vi "SmoothPath.vi"(9 "enemy_robots":T1[](array[typedef]), 10 "Path":dbl[][](array[numeric])) -> (2 "SmoothPath":dbl[][](array[numeric]))   [LabVIEW 2016]
uses:
  Core/AI Robot.ctl
  Intel/Functions Enum.ctl
  Intel/AttackerStates.ctl
  <vilib>/Analysis/_algsub.llb/Real Vector Norm.vi
  <vilib>/Analysis/baseanly.llb/Real Dot Product.vi
  <vilib>/Analysis/NI_AALBase.lvlib
  <vilib>/Analysis/NI_AALPro.lvlib
panel:
  out "y":dbl
  out "x":dbl
  out "Goal":dbl[](array[numeric])
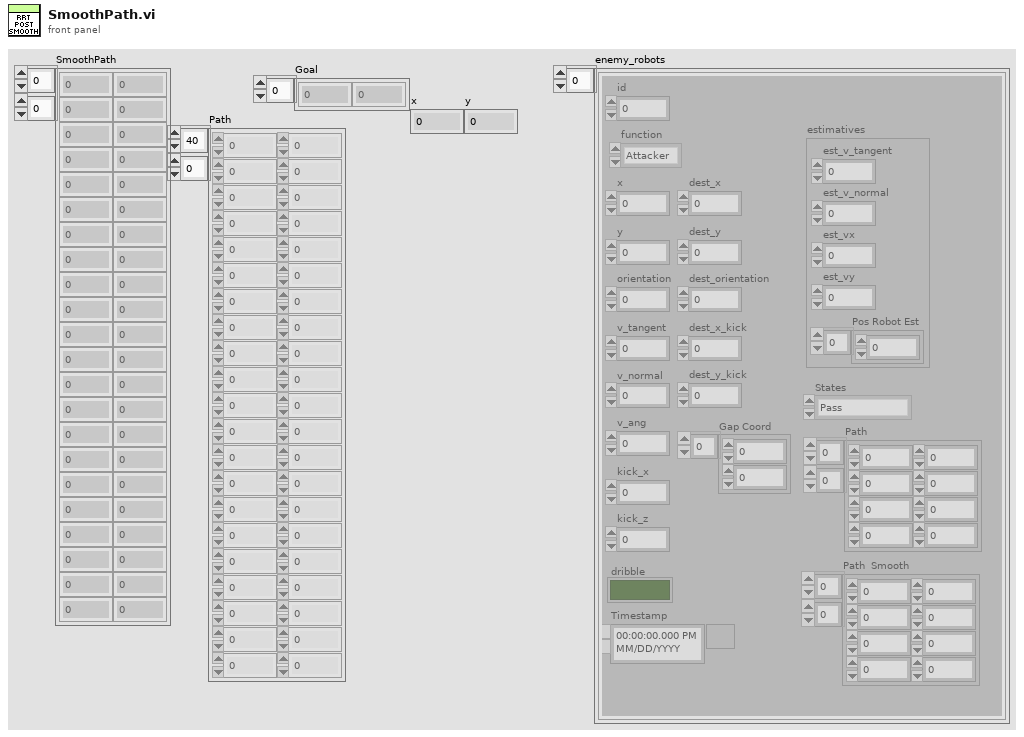
[diagram p1: front panel]
types:
  T1 = typedef "AI Robot.ctl" = cluster{"id":u32, "function":T2, "x":dbl, "y":dbl, "orientation":dbl, "v_tangent":dbl, "v_normal":dbl, "v_ang":dbl, "kick_x":dbl, "kick_z":dbl, "dribble":bool, "Timestamp":timestamp, "dest_x":dbl, "dest_y":dbl, "dest_orientation":dbl, "estimatives":cluster{"est_v_tangent":dbl, "est_v_normal":dbl, "est_vx":dbl, "est_vy":dbl, "Pos Robot Est":dbl[]}, "dest_x_kick":dbl, "dest_y_kick":dbl, "Gap Coord":dbl[], "States":T3, "Path ":dbl[][], "Path  Smooth":dbl[][]}
  T2 = typedef "Functions Enum.ctl" = enum16{"Attacker", "Goalie", "Defender", "Striker", "Goto 0", "Dummy", "Kicker", "ZigZag"}
  T3 = typedef "AttackerStates.ctl" = enum16{"Pass", "GoToTangent", "BallGetting", "GoToKick", ""}
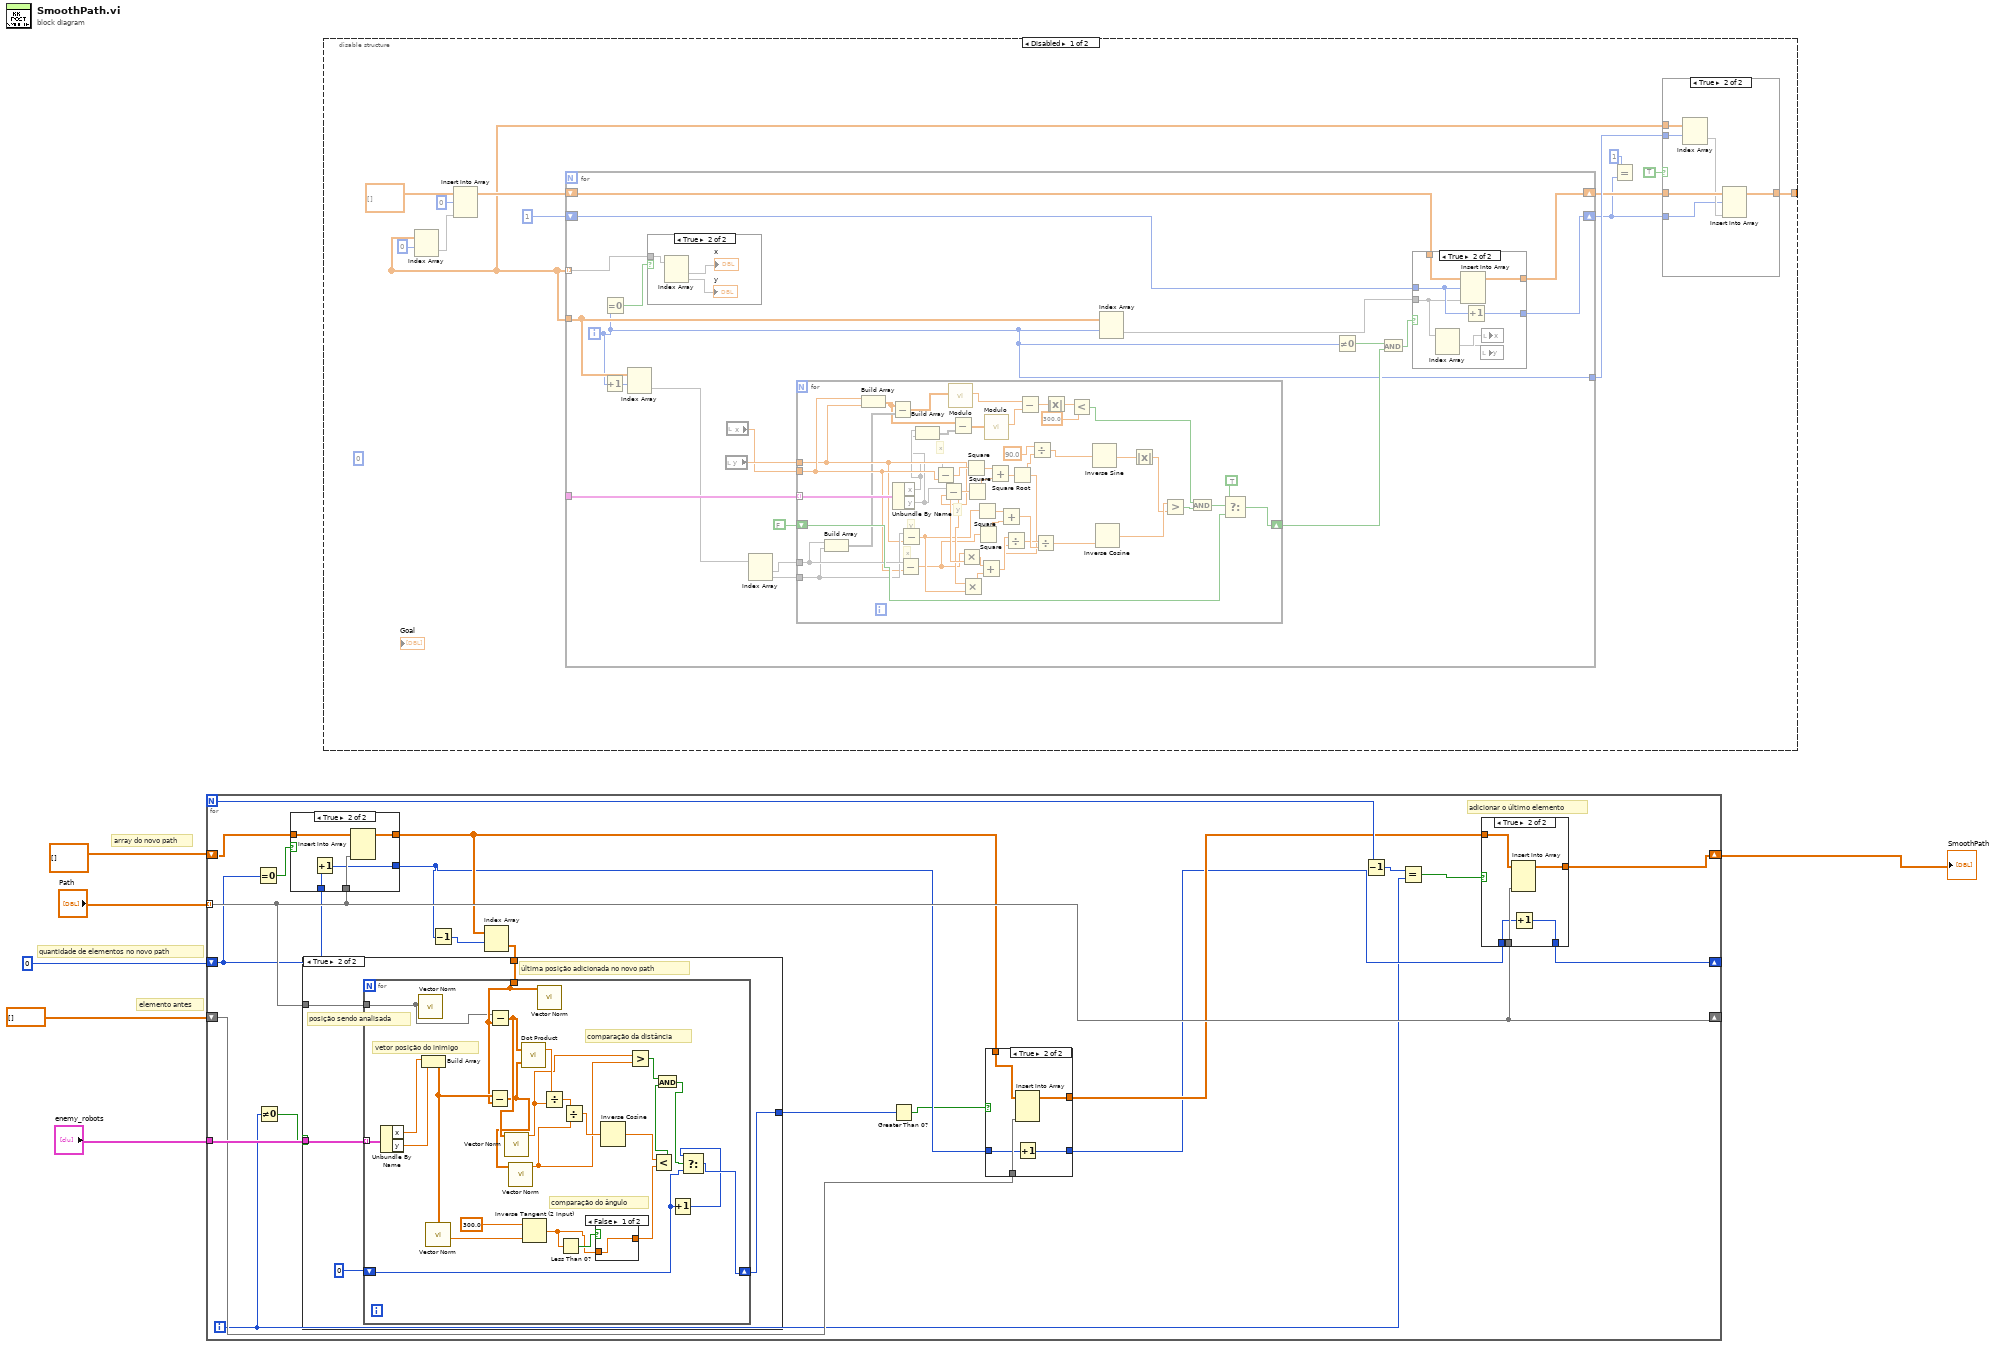
[diagram p0: block diagram]
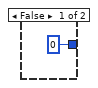
[diagram p2: hidden frame]
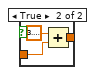
[diagram p3: hidden frame]
diagram:
  # "quantidade de elementos no novo path"
  # "elemento antes"
  # "array do novo path"
  n1 = for {
    N -> [w24]
    tunnel: "Path" -> [w22] mode=indexing
    tunnel: "enemy_robots" -> [w27]
    shift-right: [w17] -> w1
    shift-left: dbl[][] [] ("Path") -> [w21]
    shift-right: [w22] -> _
    shift-left: dbl[] [] ("Path") -> [w11]
    shift-right: [w16] -> _
    shift-left: 0 -> [w20]
    i -> [w7]
    # "adicionar o último elemento"
    n2 = Equal To 0?(x=w20) -> (x = 0?=w23:bool)
    n3 = Not Equal To 0?(x=w7) -> (x != 0?=w8:bool)
    n4 = case shown="True" w23 {
      tunnel: w22 -> [_ w76]
      tunnel: w21 -> [w70 w75]
      tunnel: [w70 w74] -> w15
      tunnel: w20 -> [w71 w73]
      tunnel: [w71 w72] -> w13
      frame False {
      }
      frame True {
        n5 = Increment(x=w73) -> (x+1=w72:i32)
        n6 = Insert Into Array(array=w75, new element=w76) -> (w74:dbl[][])  [unwired: 2 in]
      }
    }
    n7 = Decrement(x=w13) -> (x-1=w19:i32)
    n8 = Index Array(array=w15, index (row)=w19) -> (element=w18:dbl[])  [unwired: 1 in]
    n9 = case shown="True" w8 {
      tunnel: w27 -> [_ w33]
      tunnel: w22 -> [_ w31]
      tunnel: w18 -> [_ w30]
      tunnel: [0 w29] -> w10
      frame False {
      }
      frame True {
        # "última posição adicionada no novo path"
        # "posição sendo analisada"
        n10 = for {
          tunnel: w33 -> [w58] mode=indexing
          shift-right: [w44] -> w29
          shift-left: 0 -> [w42]
          tunnel: w31 -> [w51]
          tunnel: w30 -> [w52]
          # "comparação do ângulo"
          # "comparação da distância"
          # "vetor posição do inimigo"
          n11 = Unbundle By Name(w58) -> ("x"=w57:dbl, "y"=w56:dbl)
          n12 = call-poly <vilib>:"Vector Norm.vi"("Input Vector"=w51) -> ()  [unwired: 9 in, 2 out]
          n13 = Build Array(w57, w56) -> (w53:dbl[])
          n14 = call-poly <vilib>:"Vector Norm.vi"("Input Vector"=w53) -> ("norm"=w55:dbl)  [unwired: 9 in, 1 out]
          n15 = Subtract(x=w53, y=w52) -> (x-y=w45:dbl[])
          n16 = Subtract(x=w51, y=w52) -> (x-y=w49:dbl[])
          n17 = call-poly <vilib>:"Vector Norm.vi"("Input Vector"=w49) -> ("norm"=w41:dbl)  [unwired: 9 in, 1 out]
          n18 = call-poly <vilib>:"Vector Norm.vi"("Input Vector"=w45) -> ("norm"=w40:dbl)  [unwired: 9 in, 1 out]
          n19 = call-poly <vilib>:"Dot Product.vi"("Y Vector"=w45, "X Vector"=w49) -> ("X * Y"=w50:dbl)  [unwired: 1 out]
          n20 = Inverse Tangent (2 Input)(1:w55, 2:300.0 ("y")) -> (0:w35:dbl)
          n21 = call-poly <vilib>:"Vector Norm.vi"("Input Vector"=w52) -> ()  [unwired: 9 in, 2 out]
          n22 = Divide(x=w50, y=w41) -> (x/y=w48:dbl)
          n23 = Less Than 0?(x=w35) -> (x < 0?=w36:bool)
          n24 = Divide(x=w48, y=w40) -> (x/y=w47:dbl)
          n25 = case shown="False" w36 {
            tunnel: w35 -> [w59 w61]
            tunnel: [w59 w60] -> w34
            frame False {
            }
            frame True {
              n26 = Add(x=3.141592653589793, y=w61) -> (x+y=w60:dbl)
            }
          }
          n27 = Inverse Cosine(1:w47) -> (0:w46:dbl)
          n28 = Greater?(x=w41, y=w40) -> (0:w39:bool)
          n29 = Less?(x=w46, y=w34) -> (x < y?=w38:bool)
          n30 = And(x=w39, y=w38) -> (x .and. y?=w37:bool)
          n31 = Increment(x=w42) -> (x+1=w43:i32)
          n32 = Select(t=w43, s=w37, f=w42) -> (s? t:f=w44:i32)
        }
      }
    }
    n33 = Greater Than 0?(x=w10) -> (x > 0?=w9:bool)
    n34 = case shown="True" w9 {
      tunnel: w11 -> [_ w69]
      tunnel: [w63 w68] -> w14
      tunnel: w15 -> [w63 w67]
      tunnel: w13 -> [w64 w66]
      tunnel: [w64 w65] -> w12
      frame False {
      }
      frame True {
        n35 = Insert Into Array(array=w67, new element=w69) -> (w68:dbl[][])  [unwired: 2 in]
        n36 = Increment(x=w66) -> (x+1=w65:i32)
      }
    }
    n37 = Decrement(x=w24) -> (x-1=w25:i32)
    n38 = Equal?(x=w25, y=w7) -> (x = y?=w26:bool)
    n39 = case shown="True" w26 {
      tunnel: w22 -> [_ w83]
      tunnel: w14 -> [w78 w82]
      tunnel: [w78 w81] -> w17
      tunnel: w12 -> [w77 w80]
      tunnel: [w77 w79] -> w16
      frame False {
      }
      frame True {
        n40 = Insert Into Array(array=w82, new element=w83) -> (w81:dbl[][])  [unwired: 2 in]
        n41 = Increment(x=w80) -> (x+1=w79:i32)
      }
    }
  }
  "SmoothPath" <- w1
  n42 = disable-structure shown="Disabled" {
    disable-tunnel: [w87 _] -> _
    frame Disabled {
      (unwired) 0 ("index (row)")
      n43 = Index Array(array=w90, index (row)=0) -> (element=w94)  [unwired: 1 in]
      n44 = Insert Into Array(array=dbl[][] [] ("Path"), index (row)=0, new element=w94) -> (w95:dbl[][])  [unwired: 1 in]
      n45 = for {
        tunnel: [w115] -> w90 mode=indexing
        tunnel: [w124] -> w97
        shift-right: [w114] -> w88
        shift-left: w95 -> [w117]
        shift-right: [w113] -> w86
        shift-left: 1 ("index (row)") -> [w116]
        tunnel: w90 -> [w111]
        tunnel: [w105] -> w89
        i -> [w105]
        n46 = Increment(x=w105) -> (x+1=w110:i32)
        n47 = Equal To 0?(x=w105) -> (x = 0?=w123:bool)
        n48 = Index Array(array=w111, index (row)=w110) -> (element=w109)  [unwired: 1 in]
        n49 = case shown="True" w123 {
          tunnel: w115 -> [_ w136]
          frame False {
          }
          frame True {
            n50 = Index Array(array=w136) -> (element #1=→"x", element #2=→"y")  [unwired: 2 in]
          }
        }
        n51 = local read "y"() -> (w122:dbl)
        n52 = local read "x"() -> (w120:dbl)
        n53 = Index Array(array=w109) -> (element #1=w121, element #2=w119)  [unwired: 2 in]
        n54 = for {
          tunnel: w124 -> [w180] mode=indexing
          tunnel: w120 -> [w153]
          tunnel: w122 -> [w152]
          tunnel: w121 -> [w155]
          tunnel: w119 -> [w154]
          shift-right: [w160] -> w108
          shift-left: FALSE -> [w159]
          # "y"
          # "x"
          # "y"
          # "x"
          n55 = Build Array(w155, w154) -> (w151:void[])
          n56 = Build Array(w153, w152) -> (w147:dbl[])
          n57 = Subtract(x=w147, y=w151) -> (x-y=w150:dbl[])
          n58 = Unbundle By Name(w180) -> ("x"=w149, "y"=w148)
          n59 = Subtract(x=w155, y=w153) -> (x-y=w167:dbl)
          n60 = Subtract(x=w154, y=w152) -> (x-y=w168:dbl)
          n61 = Build Array(w149, w148) -> (w146:void[])
          n62 = Subtract(x=w149, y=w153) -> (x-y=w175:dbl)
          n63 = Subtract(x=w148, y=w152) -> (x-y=w174:dbl)
          n64 = call "Modulo.vi"("2D vector"=w150) -> ("Modulo"=w144:dbl)  [unwired: 10 in]
          n65 = Subtract(x=w147, y=w146) -> (x-y=w145:dbl[])
          n66 = Multiply(x=w167, y=w175) -> (x*y=w173:dbl)
          n67 = Multiply(x=w174, y=w168) -> (x*y=w172:dbl)
          n68 = Square(x=w175) -> (x^2=w179:dbl)
          n69 = Square(x=w174) -> (x^2=w178:dbl)
          n70 = Square(x=w168) -> (x^2=w170:dbl)
          n71 = Square(x=w167) -> (x^2=w169:dbl)
          n72 = Add(x=w173, y=w172) -> (x+y=w171:dbl)
          n73 = call "Modulo.vi"("2D vector"=w145) -> ("Modulo"=w143:dbl)  [unwired: 10 in]
          n74 = Add(x=w179, y=w178) -> (x+y=w177:dbl)
          n75 = Add(x=w170, y=w169) -> (x+y=w166:dbl)
          n76 = Square Root(x=w177) -> (sqrt(x)=w157:dbl)
          n77 = Divide(x=w171, y=w157) -> (x/y=w165:dbl)
          n78 = Subtract(x=w144, y=w143) -> (x-y=w142:dbl)
          n79 = Divide(x=90.0 ("y"), y=w157) -> (x/y=w176:dbl)
          n80 = Divide(x=w165, y=w166) -> (x/y=w164:dbl)
          n81 = Absolute Value(x=w142) -> (abs(x)=w141:dbl)
          n82 = Less?(x=w141, y=300.0) -> (x < y?=w137:bool)
          n83 = Inverse Sine(1:w176) -> (0:w163:dbl)
          n84 = Inverse Cosine(1:w164) -> (0:w162:dbl)
          n85 = Absolute Value(x=w163) -> (abs(x)=w161:dbl)
          n86 = Greater?(x=w162, y=w161) -> (0:w138:bool)
          n87 = And(x=w137, y=w138) -> (x .and. y?=w139:bool)
          n88 = Select(t=TRUE, s=w139, f=w159) -> (s? t:f=w160:bool)
        }
        n89 = Index Array(array=w111, index (row)=w105) -> (element=w112)  [unwired: 1 in]
        n90 = Not Equal To 0?(x=w105) -> (x != 0?=w106:bool)
        n91 = And(x=w106, y=w108) -> (x .and. y?=w107:bool)
        n92 = case shown="True" w107 {
          tunnel: w117 -> [w126 w133]
          tunnel: w116 -> [w125 w131]
          tunnel: w112 -> [_ w129]
          tunnel: [w126 w132] -> w114
          tunnel: [w125 w130] -> w113
          frame False {
          }
          frame True {
            n93 = Index Array(array=w129) -> (element #1=w128, element #2=w127)  [unwired: 2 in]
            n94 = Insert Into Array(array=w133, index (row)=w131, new element=w129) -> (w132:dbl[][])  [unwired: 1 in]
            n95 = Increment(x=w131) -> (x+1=w130:i32)
            n96 = local write "y"(w127) -> ()
            n97 = local write "x"(w128) -> ()
          }
        }
      }
      n98 = Equal?(x=1, y=w86) -> ()  [unwired: 1 out]
      n99 = case shown="True" TRUE {
        tunnel: w90 -> [_ w104]
        tunnel: w89 -> [_ w103]
        tunnel: w88 -> [w98 w102]
        tunnel: [w98 w101] -> w87
        tunnel: w86 -> [_ w99]
        frame False {
        }
        frame True {
          n100 = Index Array(array=w104, index (row)=w103) -> (element=w100)  [unwired: 1 in]
          n101 = Insert Into Array(array=w102, index (row)=w99, new element=w100) -> (w101:dbl[][])  [unwired: 1 in]
        }
      }
    }
    frame Enabled {
    }
  }
